vi "wrap.ReadOutputBuffer.vi"(0 "class.GLue in":refnum<class "class.GLue.lvclass">, 11 "error in (no error)":errorcluster) -> (4 "class.GLue out":refnum<class "class.GLue.lvclass">, 8 "String":string, 15 "error out":errorcluster)   [LabVIEW 2014, in "GLue.lvlib" / "class.GLue.lvclass"]
uses:
  class.GLue.lvclass
  class.GLue.lvclass/class.GLue.ctl
  Resources/GLue.dll
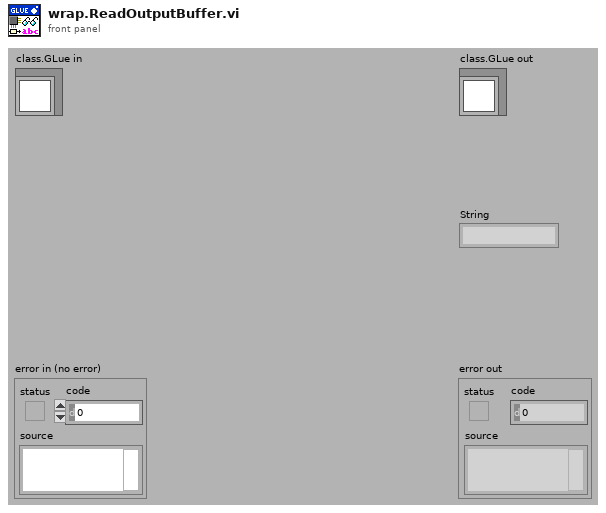
[diagram p1: front panel]
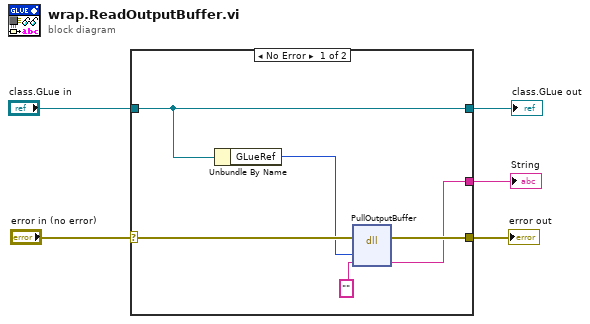
[diagram p0: block diagram]
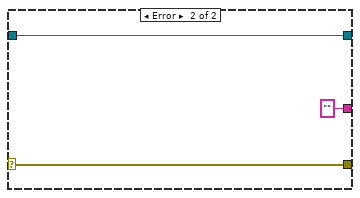
[diagram p2: hidden frame]
diagram:
  n1 = case shown="No Error" "error in (no error)" {
    selector: "error in (no error)" -> [w10 w14]
    tunnel: [w9 w14] -> w4
    tunnel: [w11 w13] -> w2
    tunnel: "class.GLue in" -> [w11 w13]
    tunnel: [w7 "" ("String")] -> w1
    frame No Error {
      n2 = Unbundle By Name(w11) -> ("GLueRef"=w8:i64)
      n3 = dll-call lib="C:/Users/Antonie/Documents/work/glue/trunk/Resources/GLue.dll" fn="PullOutputBuffer"(error in=w10, "MLua"=w8, "String"="") -> (error out=w9:errorcluster, "String"=w7:string)  [unwired: 4 in, 1 out]
    }
    frame Error {
    }
  }
  "error out" <- w4
  "class.GLue out" <- w2
  "String" <- w1
